vi "PositionVideo.vi"() -> ()   [LabVIEW 2012]
uses:
  <userlib>/_OpenG.lib/array/array.llb/Empty 1D Array (DBL)__ogtk.vi
panel:
  in  "LabVIEW file?":bool
  in  "Mode?":enum16{"Overlay", "Extend"}(ring)
  in  "Interframe time (s)":dbl
  in  "Image file pattern":string="*tif*"
  out "error out":errorcluster
  in  "error in (no error)":errorcluster
  in  "Positions file":path
  in  "Output images folder":path
  in  "Input images folder":path
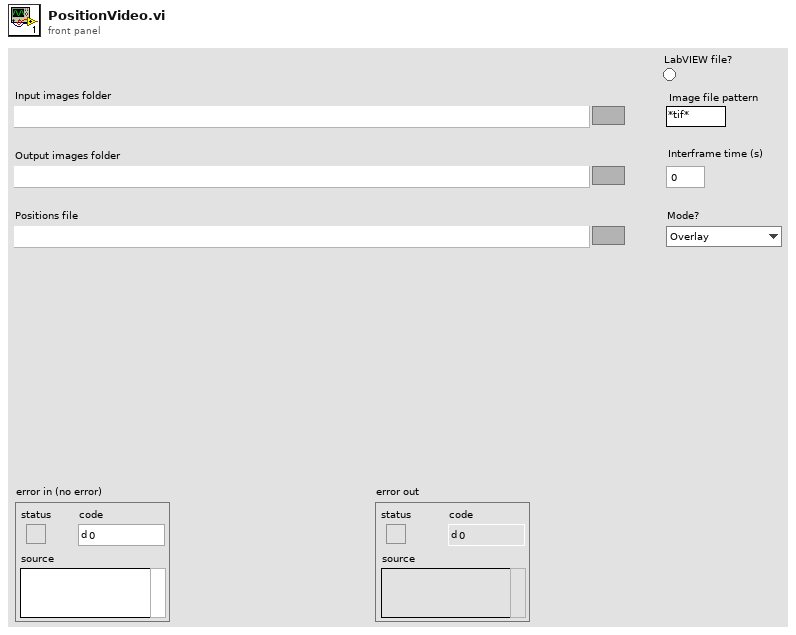
[diagram p1: front panel]
types:
  T1 = typedef "IMAQ Image.ctl" = refnum<image>
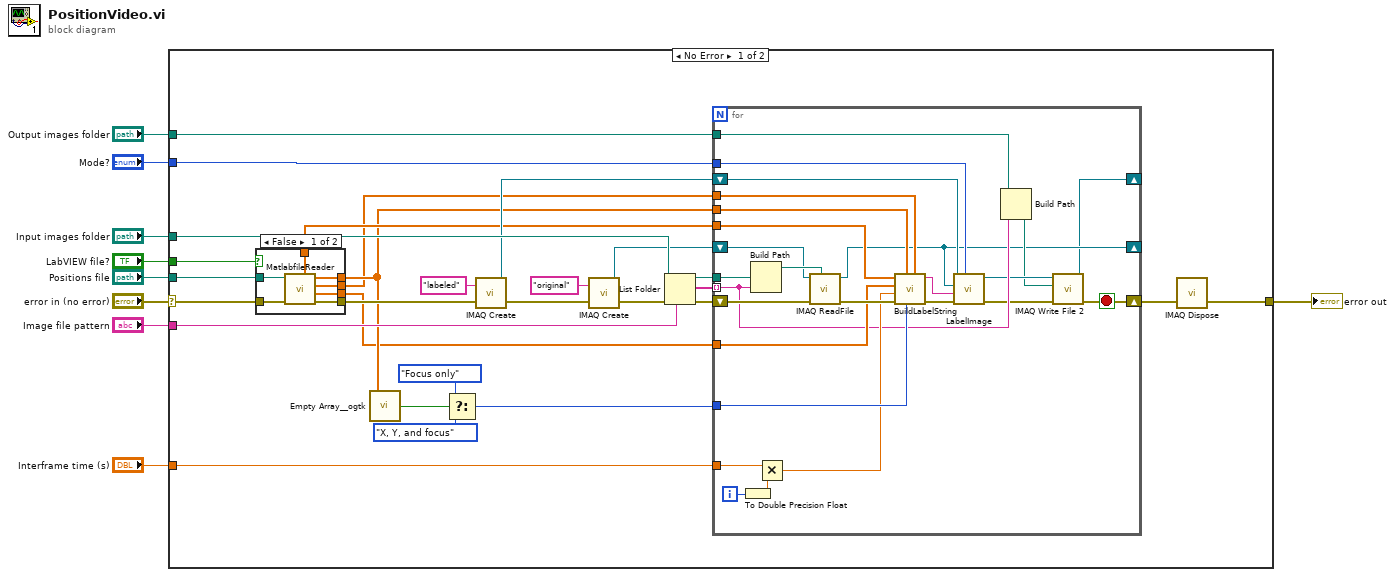
[diagram p0: block diagram]
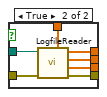
[diagram p2: hidden frame]
diagram:
  n1 = case shown="No Error" "error in (no error)" {
    selector: "error in (no error)" -> [w32 w78]
    tunnel: [w11 w78] -> w8
    tunnel: "Input images folder" -> [w37 _]
    tunnel: "Image file pattern" -> [w36 _]
    tunnel: "Positions file" -> [w31 _]
    tunnel: "Interframe time (s)" -> [w15 _]
    tunnel: "Mode?" -> [w14 _]
    tunnel: "Output images folder" -> [w13 _]
    tunnel: "LabVIEW file?" -> [w10 _]
    frame No Error {
      n2 = case shown="False" w10 {
        tunnel: w32 -> [w44 w51]
        tunnel: w31 -> [w43 w50]
        tunnel: [w42 w49] -> w29
        tunnel: [w40 w48] -> w19
        tunnel: [w39 w47] -> w18
        tunnel: [w38 w46] -> w17
        tunnel: [w41 w45] -> w16
        frame False {
          n3 = call "MatlabfileReader.vi"("error in (no error)"=w44, "Positions file"=w43) -> ("error out"=w42:errorcluster, "Focus"=w41:dbl[], "Y"=w38:dbl[], "X"=w39:dbl[], "Time"=w40:dbl[])  [unwired: 5 in]
        }
        frame True {
          n4 = call "LogfileReader.vi"("error in (no error)"=w51, "Positions file"=w50) -> ("error out"=w49:errorcluster, "Focus"=w45:dbl[], "Y"=w46:dbl[], "X"=w47:dbl[], "Time"=w48:dbl[])  [unwired: 5 in]
        }
      }
      n5 = call-poly <userlib>:"Empty Array__ogtk.vi"("Array"=w18) -> ("Empty Array?"=w22:bool)  [unwired: 8 in]
      n6 = Select(t=enum16{"Focus only", "X, Y, and focus"}."Focus only" ("Axes"), s=w22, f=enum16{"Focus only", "X, Y, and focus"}."X, Y, and focus" ("Axes")) -> (s? t:f=w20:enum16{"Focus only", "X, Y, and focus"})
      n7 = call "IMAQ Create"("Image Name"="labeled", "error in (no error)"=w29) -> ("New Image"=w25:T1, "error out"=w30:errorcluster)  [unwired: 3 in]
      n8 = call "IMAQ Create"("Image Name"="original", "error in (no error)"=w30) -> ("New Image"=w24:T1, "error out"=w28:errorcluster)  [unwired: 3 in]
      n9 = List Folder(path=w37, pattern=w36, error in=w28) -> (path out=w34:path, filenames=w33:string[], error out=w35:errorcluster)  [unwired: 1 in, 1 out]
      n10 = for {
        shift-right: [w52] -> w12
        shift-left: w35 -> [w76]
        tunnel: w34 -> [w77]
        tunnel: w33 -> [w58] mode=indexing
        tunnel: w20 -> [w73]
        tunnel: w19 -> [w70]
        tunnel: w18 -> [w69]
        tunnel: w17 -> [w68]
        tunnel: w16 -> [w67]
        tunnel: w15 -> [w64]
        tunnel: w14 -> [w60]
        tunnel: w13 -> [w59]
        shift-right: [w53] -> _
        shift-left: w25 -> [w61]
        shift-right: [w54] -> _
        shift-left: w24 -> [w74]
        i -> [w66]
        stop <- w52 stop-if-true
        n11 = To Double Precision Float(number=w66) -> (double precision float=w65:dbl)
        n12 = Build Path(base path=w77, name or relative path=w58) -> (appended path=w75:path)
        n13 = Multiply(x=w64, y=w65) -> (x*y=w63:dbl)
        n14 = call "IMAQ ReadFile"("File Path"=w75, "error in (no error)"=w76, "Image"=w74) -> ("error out"=w72:errorcluster, "Image Out"=w54:T1)  [unwired: 4 in, 3 out]
        n15 = call "BuildLabelString.vi"("Y"=w68, "Axes"=w73, "X"=w69, "error in (no error)"=w72, "Image time"=w63, "Focus"=w67, "Time array"=w70) -> ("error out"=w71:errorcluster, "Label string"=w62:string)  [unwired: 3 in]
        n16 = call "LabelImage.vi"("Mode?"=w60, "error in (no error)"=w71, "Label"=w62, "Original image in"=w54, "Labeled image in"=w61) -> ("error out"=w57:errorcluster, "Labeled image out"=w56:T1)  [unwired: 4 in, 1 out]
        n17 = Build Path(base path=w59, name or relative path=w58) -> (appended path=w55:path)
        n18 = call-poly "IMAQ Write File 2"("error in (no error)"=w57, "File Path"=w55, "Image"=w56) -> ("error out"=w52:errorcluster, "Image Out (duplicate)"=w53:T1)  [unwired: 7 in]
      }
      n19 = call "IMAQ Dispose"("error in (no error)"=w12) -> ("error out"=w11:errorcluster)  [unwired: 5 in]
    }
    frame Error {
    }
  }
  "error out" <- w8
